vi "Get Fixed-Point Raw Data.vi"(8 "Error In":errorcluster) -> (0 "error out":errorcluster, 1 "Values":dbl[](array[numeric]))   [LabVIEW 2018]
uses:
  NiFpga.dll
panel:
  out "status":i32
  out "Read + Convert Graph":dbl[](graph)
  out "Read Graph":dbl[](graph)
  out "Read + Convert Average":dbl
  out "Read Average":dbl
  out "FXP Value":dbl
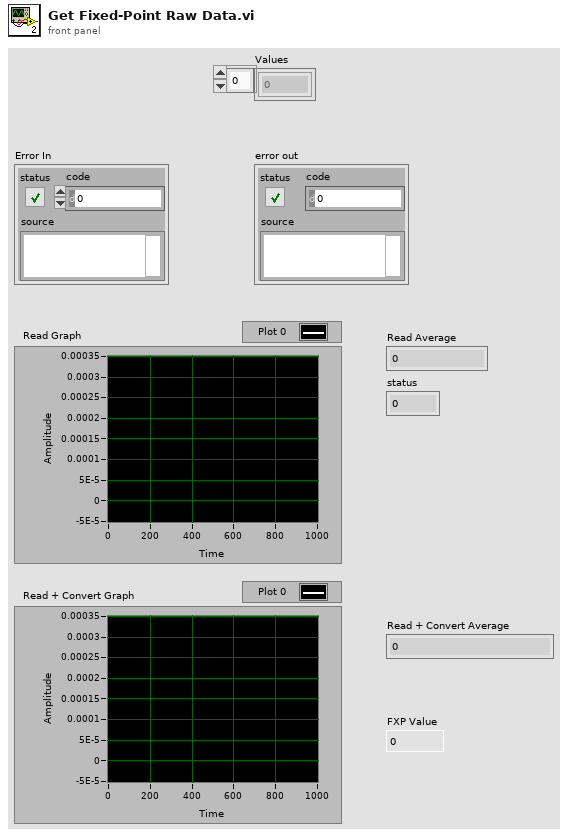
[diagram p1: front panel]
types:
  T1 = cluster{"Delta":dbl, "Word Length":i8, "Signed":bool, "offset":i32, "Name":string, "base address":i32}[]
  T2 = cluster{"Delta":dbl, "Word Length":i8, "Signed":bool, "offset":i32, "Name":string, "base address":i32}
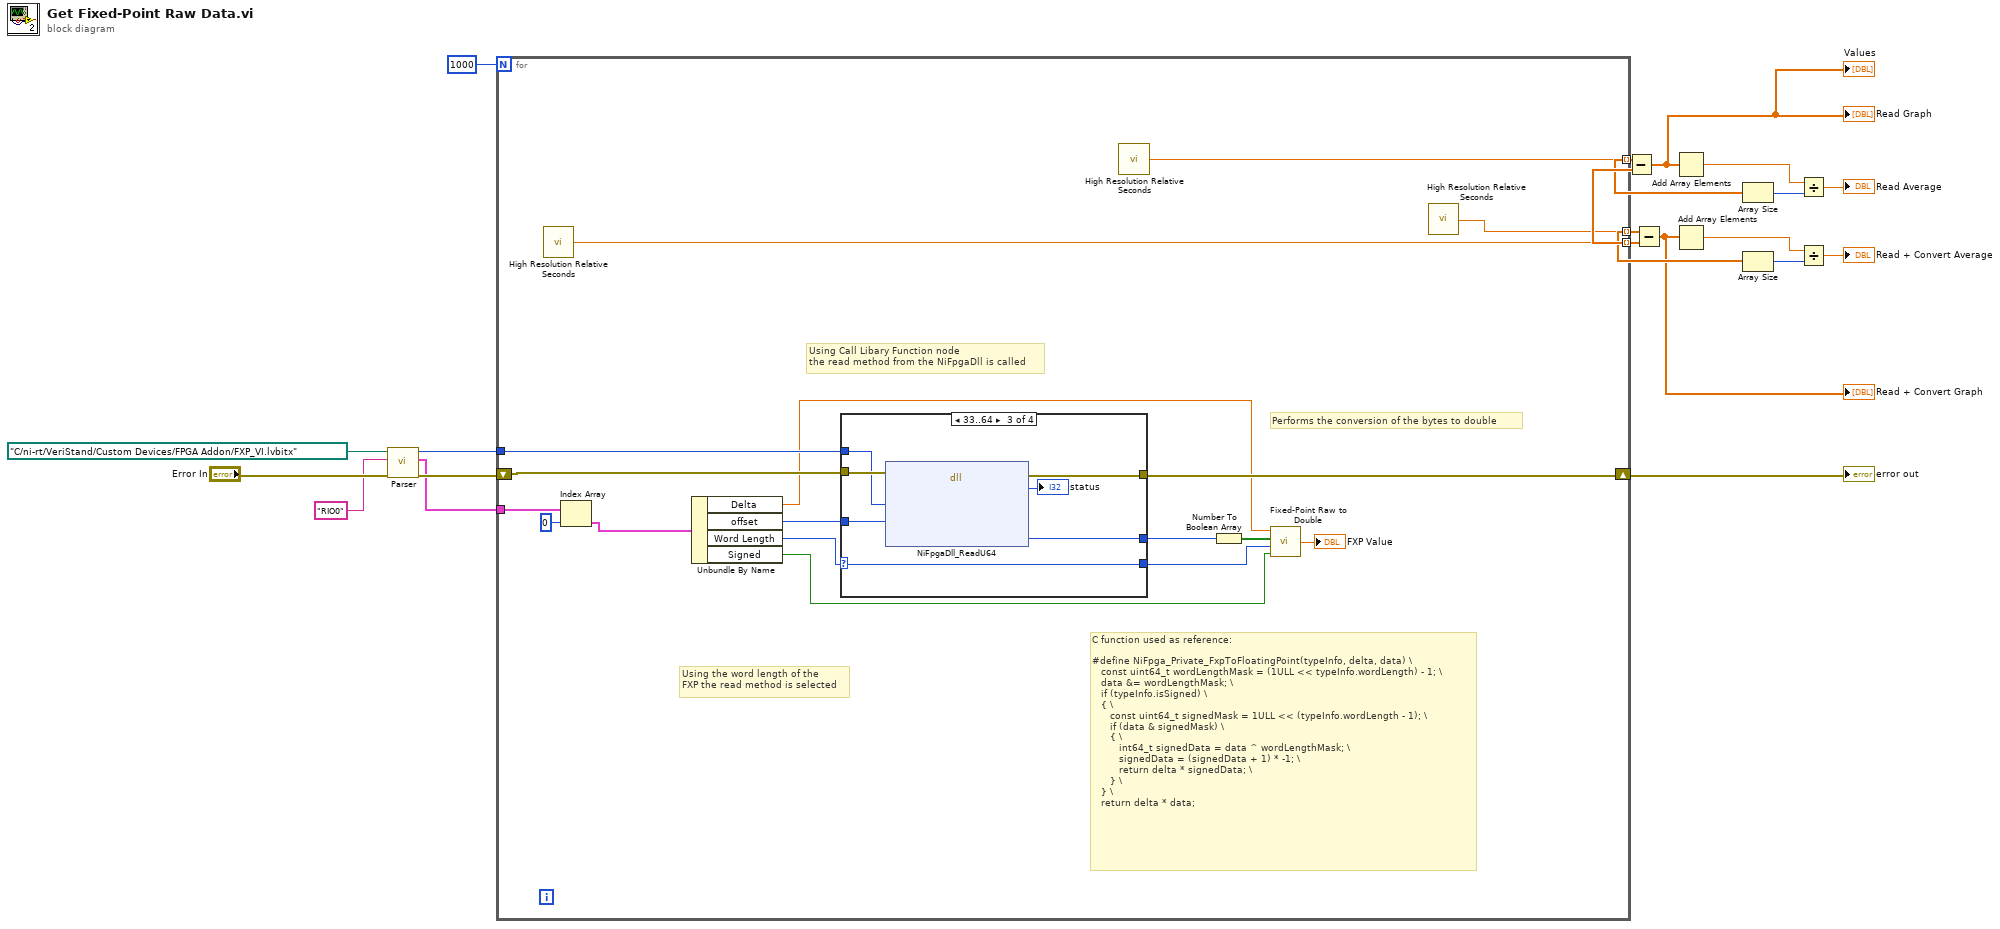
[diagram p0: block diagram]
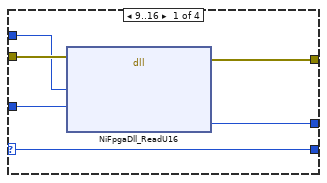
[diagram p2: hidden frame]
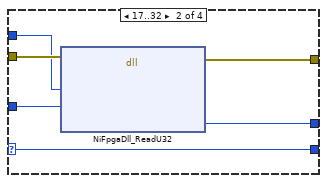
[diagram p3: hidden frame]
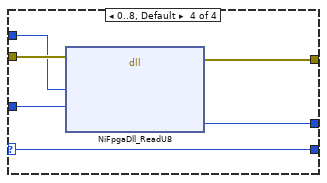
[diagram p4: hidden frame]
diagram:
  n1 = call "Parser.vi"("error in (no error)"="Error In", "RIO device address"="RIO0" ("Device address"), "bitfile path"=path "C:/ni-rt/VeriStand/Custom Devices/FPGA Addon/FXP_VI.lvbitx" ("Bitfile path")) -> ("error out"=w17:errorcluster, "FXP channels out"=w1:T1, "session out"=w15:u64)  [unwired: 6 in]
  n2 = for {
    N: 1000 -> [_]
    tunnel: w15 -> [w34]
    shift-right: [w36] -> w6
    shift-left: w17 -> [w35]
    tunnel: [w33] -> w4 mode=indexing
    tunnel: [w30] -> w13 mode=indexing
    tunnel: [w29] -> w5 mode=indexing
    tunnel: w1 -> [w24]
    # "Performs the conversion of the bytes to double"
    # "C function used as reference:\n\n#define NiFpga_Private_FxpToFloatingPoint(typeInfo, delta, data) \\\n   const uint64_t wordLengthMask = (1ULL << typeInfo.wordLength) - 1; \\\n   data &= wordLengthMask; \\\n   if (typeInfo.isSigned) \\\n   { \\\n      const uint64_t signedMask = 1ULL << (typeInfo.wordLength - 1); \\\n      if (data & signedMask) \\\n      { \\\n         int64_t signedData = data ^ wordLengthMask; \\\n         signedData = (signedData + 1) * -1; \\\n         return delta * signedData; \\\n      } \\\n   } \\\n   return delta * data;"
    # "Using Call Libary Function node\nthe read method from the NiFpgaDll is called"
    # "Using the word length of the \nFXP the read method is selected"
    n3 = call <vilib>:"High Resolution Relative Seconds.vi"() -> ("relative seconds"=w30:dbl)
    n4 = Index Array(array=w24, index=0) -> (element=w23:T2)
    n5 = Unbundle By Name(w23) -> ("Delta"=w22:dbl, "offset"=w27:i32, "Word Length"=w20:i8, "Signed"=w21:bool)
    n6 = case shown="33..64" w20 {
      selector: w20 -> [w40 w46 w53 w59]
      tunnel: [w42 w47 w55 w61] -> w36
      tunnel: [w41 w48 w54 w60] -> w31
      tunnel: [w40 w46 w53 w59] -> w32
      tunnel: w35 -> [w39 w45 w52 w58]
      tunnel: w34 -> [w38 w44 w51 w57]
      tunnel: w27 -> [w37 w43 w50 w56]
      frame 9..16 {
        n7 = dll-call lib="NiFpga.*" fn="NiFpgaDll_ReadU16"(error in=w39, "session"=w38, "offset"=w37) -> (error out=w42:errorcluster, "value"=w41:u8)  [unwired: 6 in, 1 out]
      }
      frame 17..32 {
        n8 = dll-call lib="NiFpga.*" fn="NiFpgaDll_ReadU32"(error in=w45, "session"=w44, "offset"=w43) -> (error out=w47:errorcluster, "value"=w48:u8)  [unwired: 6 in, 1 out]
      }
      frame 33..64 {
        n9 = dll-call lib="NiFpga.*" fn="NiFpgaDll_ReadU64"(error in=w52, "session"=w51, "offset"=w50) -> (error out=w55:errorcluster, "status"=→"status":i32, "value"=w54:u8)  [unwired: 5 in, 1 out]
      }
      frame 0..8, Default {
        n10 = dll-call lib="NiFpga.*" fn="NiFpgaDll_ReadU8"(error in=w58, "session"=w57, "offset"=w56) -> (error out=w61:errorcluster, "value"=w60:u8)  [unwired: 6 in, 1 out]
      }
    }
    n11 = call <vilib>:"High Resolution Relative Seconds.vi"() -> ("relative seconds"=w29:dbl)
    n12 = Number To Boolean Array(number=w31) -> (Boolean array=w25:bool[])
    n13 = call "Fixed-Point Raw to Double.vi"("Signed?"=w21, "Word Length"=w32, "Data"=w25, "Delta"=w22) -> ("value"=→"FXP Value":dbl)
    n14 = call <vilib>:"High Resolution Relative Seconds.vi"() -> ("relative seconds"=w33:dbl)
  }
  "error out" <- w6
  n15 = Subtract(x=w5, y=w13) -> (x-y=w3:dbl[])
  "Read Graph" <- w3
  "Values" <- w3
  n16 = Subtract(x=w4, y=w13) -> (x-y=w2:dbl[])
  "Read + Convert Graph" <- w2
  n17 = Add Array Elements(numeric array=w3) -> (sum=w12:dbl)
  n18 = Add Array Elements(numeric array=w2) -> (sum=w8:dbl)
  n19 = Array Size(array=w5) -> (size(s)=w11:i32)
  n20 = Array Size(array=w4) -> (size(s)=w9:i32)
  n21 = Divide(x=w12, y=w11) -> (x/y=→"Read Average":dbl)
  n22 = Divide(x=w8, y=w9) -> (x/y=→"Read + Convert Average":dbl)
